vi "Numeric.vi"(8 "error in (no error)":errorcluster, 10 "Keys":string[](array[string]), 11 "JSON Object in":refnum<class "JSON Object.lvclass">) -> (0 "error out":errorcluster, 1 "found?":bool, 2 "JSON Datatype out":refnum<class "JSON Numeric.lvclass">)   [LabVIEW 2015, in "LVJSON.lvlib" / "JSON Object.lvclass"]
uses:
  JSON Object.lvclass
  JSON Numeric/JSON Numeric.lvclass
  JSON Datatype/To More Specific Type (Numeric).vi
  JSON Datatype/JSON Datatype.lvclass
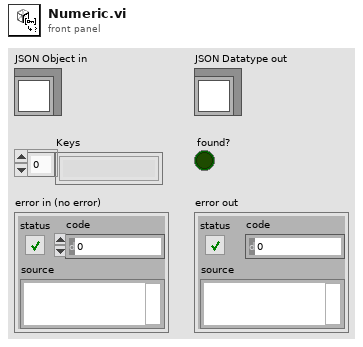
[diagram p1: front panel]
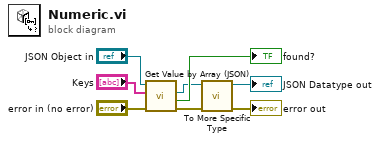
[diagram p0: block diagram]
diagram:
  n1 = call "Get Value by Array (JSON).vi"("error in (no error)"="error in (no error)", "Keys"="Keys", "JSON Object in"="JSON Object in") -> ("error out"=w4:errorcluster, "found?"=→"found?":bool, "JSON Datatype out"=w3:refnum<class "JSON Datatype.lvclass">)  [unwired: 6 in]
  n2 = call-poly "To More Specific Type.vi"("error in (no error)"=w4, "JSON Datatype in"=w3) -> ("error out"=→"error out":errorcluster, "JSON Numeric out"=→"JSON Datatype out":refnum<class "JSON Numeric.lvclass">)  [unwired: 8 in]
